vi "Read InstanceInfo.vi"(8 "error in (no error)":errorcluster, 11 "Polymorphic VI Type in":refnum<class "Polymorphic VI Type.lvclass">) -> (0 "error out":errorcluster, 2 "InstanceInfo":T1(array[cluster]), 3 "Polymorphic VI Type out":refnum<class "Polymorphic VI Type.lvclass">)   [LabVIEW 2020, in "Peek Window.lvlib" / "Polymorphic VI Type.lvclass"]
doc: "Basic read acceessor."
uses:
  Polymorphic VI Type.lvclass
  Polymorphic VI Type.lvclass/Polymorphic VI Type.ctl
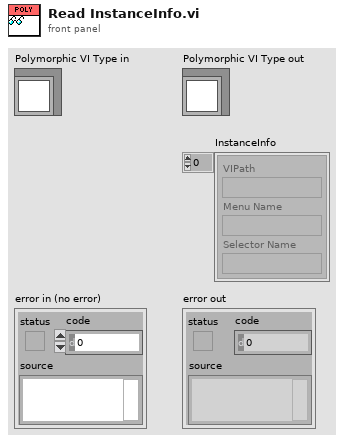
[diagram p1: front panel]
types:
  T1 = cluster{"VIPath":path, "Menu Name":string, "Selector Name":string}[]
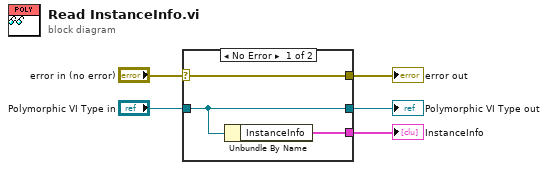
[diagram p0: block diagram]
diagram:
  n1 = case shown="No Error" "error in (no error)" {
    selector: "error in (no error)" -> [w8 w9]
    tunnel: [w8 w9] -> w4
    tunnel: [w7 w10] -> w2
    tunnel: "Polymorphic VI Type in" -> [w7 w10]
    tunnel: [w6 _] -> w1
    frame No Error {
      n2 = Unbundle By Name(w7) -> ("InstanceInfo"=w6:T1)
    }
    frame Error {
    }
  }
  "error out" <- w4
  "Polymorphic VI Type out" <- w2
  "InstanceInfo" <- w1
